vi "odor config arr descrip update (sub-vi).vi"(8 "error in (no error)":errorcluster, 11 "array refnum":refnum<vi>) -> (0 "error out":errorcluster, 3 "array refnum out":refnum<vi>)   [LabVIEW 2021]
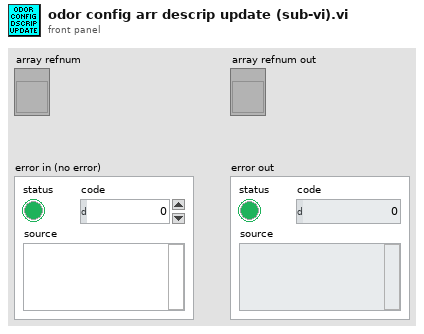
[diagram p1: front panel]
types:
  T1 = typedef "odor description array (type def).ctl" = T2[]
  T2 = typedef "odor info cluster (type def).ctl" = cluster{"odor channel":T3, "odor description":string, "odor color":T4, "odor channel active":bool}
  T3 = typedef "odor selection (type def).ctl" = enum16{"[none]", "odor 1", "odor 2", "odor 3", "odor 4", "odor 5", "odor 6", "odor 7", "odor 8", "odor 9", "odor 10"}
  T4 = typedef "odor color (type def).ctl" = u16
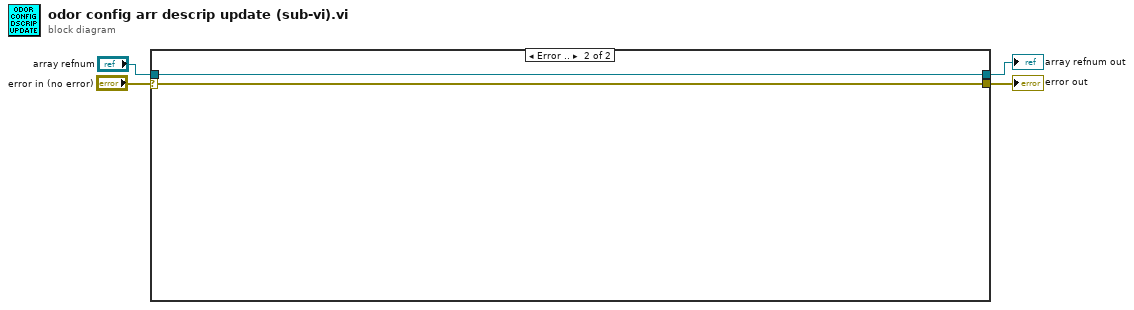
[diagram p0: block diagram]
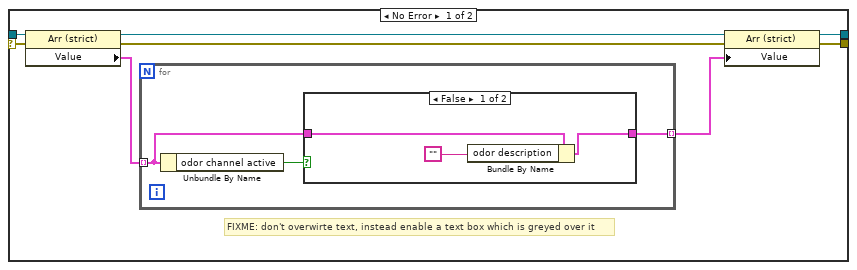
[diagram p2: hidden frame]
diagram:
  n1 = case shown="Error .." "error in (no error)" {
    selector: "error in (no error)" -> [w7 w20]
    tunnel: [w12 w20] -> w4
    tunnel: "array refnum" -> [w6 w21]
    tunnel: [w5 w21] -> w1
    frame No Error {
      # "FIXME: don't overwirte text, instead enable a text box which is greyed over it"
      n2 = property class="Arr (strict)"(reference=w6, error in=w7) -> (reference out=w11:refnum<vi>, error out=w10:errorcluster, "Value"=w8:T1)
      n3 = for {
        tunnel: w8 -> [w14] mode=indexing
        tunnel: [w13] -> w9 mode=indexing
        n4 = Unbundle By Name(w14) -> ("odor channel active"=w15:bool)
        n5 = case shown="False" w15 {
          tunnel: [w17 w19] -> w13
          tunnel: w14 -> [w18 w19]
          frame False {
            n6 = Bundle By Name(cluster=w18, "odor description"="") -> (w17:T2)
          }
          frame True {
          }
        }
      }
      n7 = property class="Arr (strict)"(reference=w11, error in=w10, "Value"=w9) -> (reference out=w5:refnum<vi>, error out=w12:errorcluster)
    }
    frame Error {
    }
  }
  "array refnum out" <- w1
  "error out" <- w4
